vi "Get Protocol Type.vi"(8 "error in (no error)":errorcluster, 11 "AK TCP in":refnum<class "AK TCP.lvclass">) -> (0 "error out":errorcluster, 2 "protocol type":T1=enum."AK RS-XXX", 3 "AK TCP out":refnum<class "AK TCP.lvclass">)   [LabVIEW 2018, in "Protocols.lvlib" / "AK TCP.lvclass"]
uses:
  AK TCP.lvclass
  Protocol Parent/Types/Protocol Type.ctl
  Protocol Parent/Protocol Parent.lvclass
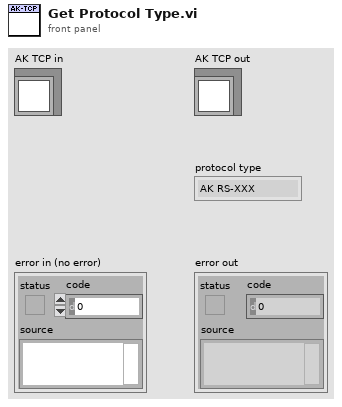
[diagram p1: front panel]
types:
  T1 = typedef "Protocols.lvlib/Protocol Parent.lvclass/Protocol Type.ctl" = enum16{"RS-XXX", "AK RS-XXX", "VISA", "TCPIP", "AK TCPIP", "UDP", "GPIB ConvBox"}
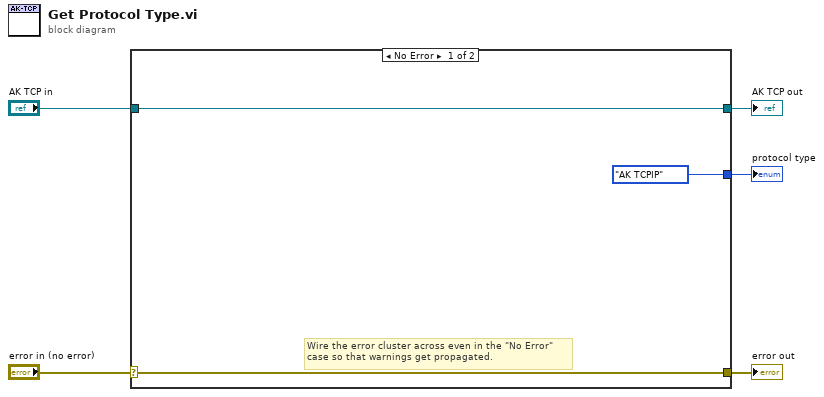
[diagram p0: block diagram]
diagram:
  n1 = case shown="No Error" "error in (no error)" {
    selector: "error in (no error)" -> [w7 w10]
    tunnel: [w7 w10] -> w4
    tunnel: [w8 w9] -> w2
    tunnel: "AK TCP in" -> [w8 w9]
    tunnel: [Protocol_Type."AK TCPIP" ("Protocol out") _] -> w1
    frame No Error {
      # "Wire the error cluster across even in the \"No Error\"\ncase so that warnings get propagated."
    }
    frame Error {
    }
  }
  "error out" <- w4
  "AK TCP out" <- w2
  "protocol type" <- w1
